vi "Get Motor Power Status_all.vi"(4 "error in (no error)":errorcluster, 5 "ESP302 in":refnum<class "ESP302.lvclass">, 7 "VISA resource name":refnum<visa-resource-name>) -> (0 "error out":errorcluster, 1 "ESP302 out":refnum<class "ESP302.lvclass">, 2 "Power Status":bool[](array[boolean]), 3 "VISA resource name out":refnum<visa-resource-name>)   [LabVIEW 2020, in "ESP302.lvclass"]
doc: "Get the power status of one axis."
uses:
  ESP302/ESP302.lvclass
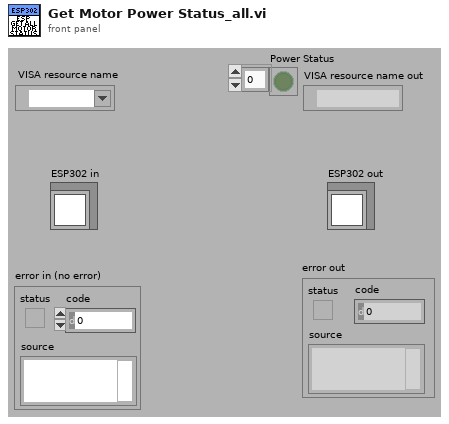
[diagram p1: front panel]
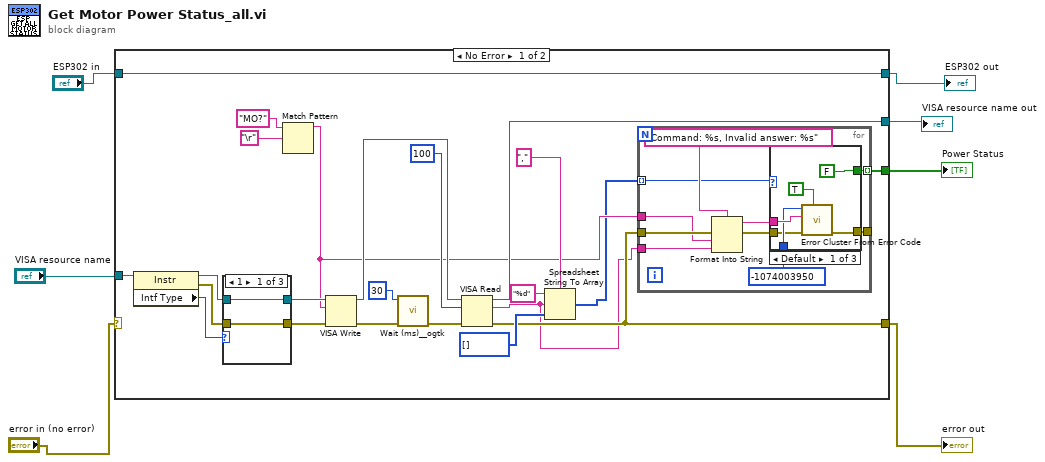
[diagram p0: block diagram]
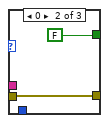
[diagram p2: hidden frame]
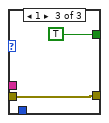
[diagram p3: hidden frame]
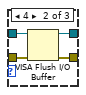
[diagram p4: hidden frame]
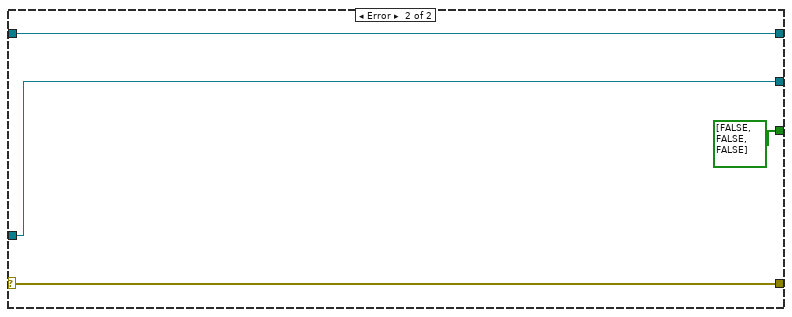
[diagram p6: hidden frame]
diagram:
  n1 = case shown="No Error" "error in (no error)" {
    selector: "error in (no error)" -> [_ w60]
    tunnel: "VISA resource name" -> [w20 w61]
    tunnel: [w12 w60] -> w3
    tunnel: [w19 w61] -> w2
    tunnel: "ESP302 in" -> [w18 w62]
    tunnel: [w18 w62] -> w6
    tunnel: [w8 bool[] [FALSE, FALSE, FALSE]] -> w4
    frame No Error {
      n2 = property class="Instr"(reference=w20) -> (reference out=w24:refnum<visa-resource-name>, error out=w23:errorcluster, "Intf Type"=w25:u16)  [unwired: 1 in]
      n3 = case shown="1" w25 {
        tunnel: w24 -> [w52 w54 w58]
        tunnel: [w52 w53 w58] -> w29
        tunnel: w23 -> [w51 w56 w57]
        tunnel: [w51 w55 w57] -> w28
        frame 1 {
        }
        frame 4 {
          n4 = VISA Flush I/O Buffer(VISA resource name=w54, error in (no error)=w56) -> (VISA resource name out=w53:refnum<visa-resource-name>, error out=w55:errorcluster)  [unwired: 1 out]
        }
        frame Default {
        }
      }
      n5 = Match Pattern(string="MO?" ("Read Actual\nPosition"), regular expression="\r") -> (before substring=w11:string)  [unwired: 4 out]
      n6 = VISA Write(VISA resource name=w29, write buffer=w11, error in (no error)=w28) -> (VISA resource name out=w30:refnum<visa-resource-name>, error out=w27:errorcluster)  [unwired: 1 out]
      n7 = call <userlib>:"Wait (ms)__ogtk.vi"("error in (no error)"=w27, "milliseconds to wait"=u32 30 ("Wait before read (0ms)")) -> ("error out"=w17:errorcluster)  [unwired: 8 in, 1 out]
      n8 = VISA Read(VISA resource name=w30, byte count=u32 100 ("Bytes to read (100)"), error in (no error)=w17) -> (VISA resource name out=w19:refnum<visa-resource-name>, read buffer=w10:string, error out=w12:errorcluster)  [unwired: 1 out]
      n9 = Spreadsheet String To Array(delimiter (Tab)=",", format string="%d", spreadsheet string=w10, array type (2D Dbl)=i32[] []) -> (array=w9:i32[])
      n10 = for {
        tunnel: w12 -> [w38]
        tunnel: [w37] -> w8 mode=indexing
        tunnel: [w34] -> _
        tunnel: w11 -> [w33]
        tunnel: w10 -> [w32]
        tunnel: w9 -> [w31] mode=indexing
        n11 = Format Into String(format string="Command: %s, Invalid answer: %s" ("error message (\"\")"), error in=w38, w33, w32) -> (resulting string=w40:string, error out=w35:errorcluster)  [unwired: 1 in]
        n12 = case shown="Default" w31 {
          tunnel: [FALSE ("Motion Done") FALSE ("Motion Done") TRUE ("Motion Done")] -> w37
          tunnel: w40 -> [w44 _ _]
          tunnel: -1074003950 ("error code (0)") -> [w43 _ _]
          tunnel: w35 -> [w42 w47 w49]
          tunnel: [w41 w47 w49] -> w34
          frame Default {
            n13 = call <vilib>:"Error Cluster From Error Code.vi"("show call chain? (False)"=TRUE, "error in (no error)"=w42, "error message (\"\")"=w44, "error code (0)"=w43) -> ("error out"=w41:errorcluster)  [unwired: 5 in]
          }
          frame 0 {
          }
          frame 1 {
          }
        }
      }
    }
    frame Error {
    }
  }
  "error out" <- w3
  "VISA resource name out" <- w2
  "Power Status" <- w4
  "ESP302 out" <- w6
